vi "Photostimulation engine.vi"(8 "external trigger enabled?":bool, 9 "waveform repetitions":dbl, 10 "pockels and piezo data in":waveform(dbl)[](array[waveform]), 11 "x-y mirror data in":waveform(dbl)[](array[waveform])) -> ()   [LabVIEW 2012]
uses:
  <vilib>/DAQmx/write.llb/DAQmx Write (Analog 1D Wfm NChan NSamp).vi
  <vilib>/Waveform/WDTOps.llb/WDT Number of Waveform Samples DBL.vi
  <vilib>/DAQmx/create/channels.llb/DAQmx Create Channel (AO-Voltage-Basic).vi
  <vilib>/DAQmx/configure/trigger.llb/DAQmx Start Trigger (Digital Edge).vi
  <vilib>/DAQmx/miscellaneous.llb/DAQmx Fill In Error Info.vi
  <resource>/objmgr/daqmx.rc
panel:
  out "String 3":string
  in  "stop 3":bool
  in  "stop 2":bool
  out "Waveform Graph 2":waveform(dbl)[](graph)
  out "Waveform Graph":waveform(dbl)[](graph)
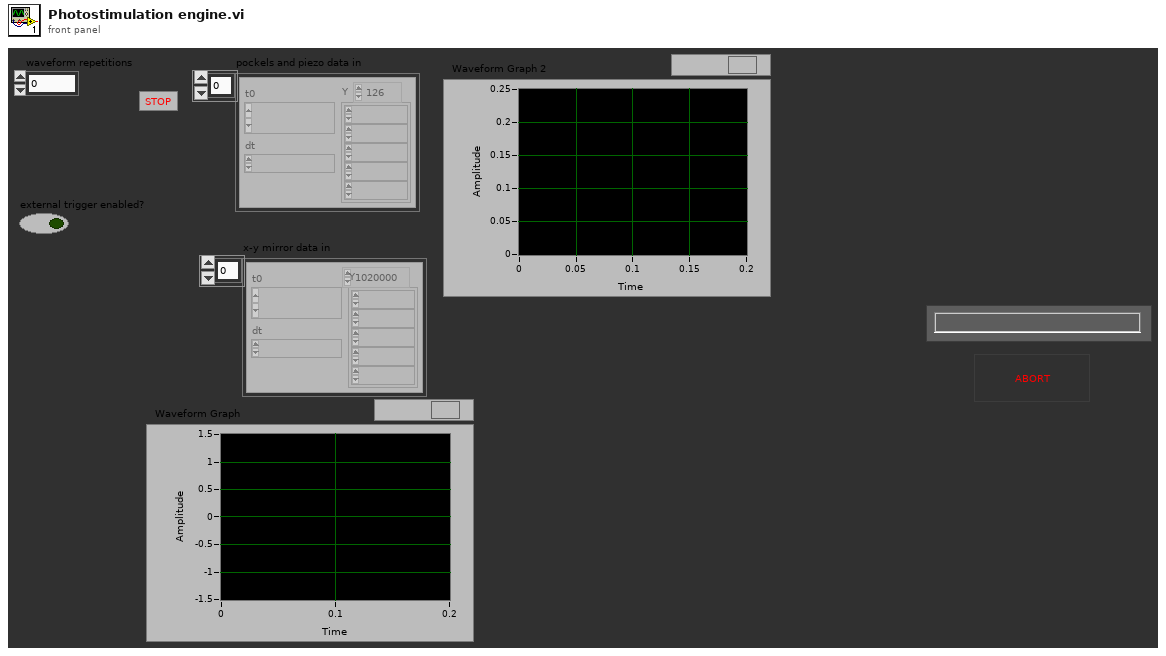
[diagram p1: front panel]
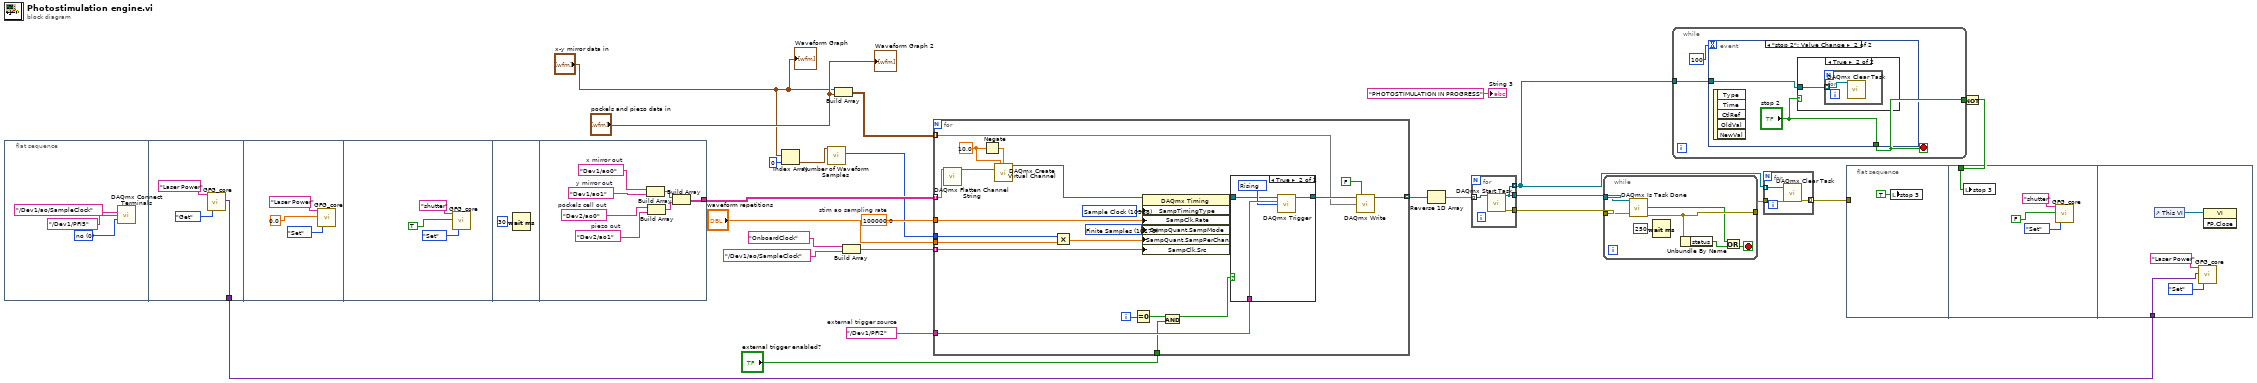
[diagram p0: block diagram]
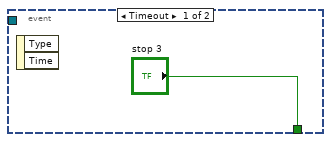
[diagram p2: hidden frame]
diagram:
  w20 = 100000.0  # stim ao sampling rate
  w17 = tag "/Dev1/PFI2"  # external trigger source
  n1 = flat-sequence {
    tunnel: [w29] -> w1
    tunnel: [w39] -> w22
    frame #0 {
      w26 = 0 items=["no", "yes"] ("invert polarity")
      n2 = call <vilib>:"DAQmx Connect Terminals.vi"("source terminal"=tag "/Dev1/ao/SampleClock", "destination terminal"=tag "/Dev1/PFI5", "invert polarity"=w26) -> ()  [unwired: 12 in, 1 out]
    }
    frame #1 {
      n3 = call "GFG_core.vi"("Variable Name in"="Laser Power", "Action"=enum16{"Init", "Set", "Get", "Clear"}."Get") -> ("Variant Out"=w29:variant)  [unwired: 11 in, 6 out]
    }
    frame #2 {
      n4 = call "GFG_core.vi"("Variable Name in"="Laser Power", "Variant in"=0.0 ("waveform repetitions"), "Action"=enum16{"Init", "Set", "Get", "Clear"}."Set") -> ()  [unwired: 10 in, 7 out]
    }
    frame #3 {
      n5 = call "GFG_core.vi"("Variable Name in"="shutter", "Variant in"=TRUE ("external trigger enabled?"), "Action"=enum16{"Init", "Set", "Get", "Clear"}."Set") -> ()  [unwired: 10 in, 7 out]
    }
    frame #4 {
      n6 = Wait (ms)(milliseconds to wait=u32 30) -> ()  [unwired: 1 out]
    }
    frame #5 {
      w42 = tag "Dev2/ao1"  # piezo out
      w43 = tag "Dev2/ao0"  # pockels cell out
      w45 = tag "Dev1/ao1"  # y mirror out
      w44 = tag "Dev1/ao0"  # x mirror out
      n7 = Build Array(w44, w45) -> (w40:tag[])
      n8 = Build Array(w43, w42) -> (w41:tag[])
      n9 = Build Array(w40, w41) -> (w39:tag[][])
    }
  }
  n10 = Index Array(array="x-y mirror data in", index=0) -> (element=w10:waveform(dbl))
  n11 = call-poly <vilib>:"Number of Waveform Samples.vi"("waveform in"=w10) -> ("number of samples"=w9:i32)  [unwired: 8 in, 2 out]
  n12 = Build Array("x-y mirror data in", "pockels and piezo data in") -> (w21:waveform(dbl)[][])
  n13 = Build Array(tag "OnboardClock" ("SampClk.Src"), tag "/Dev1/ao/SampleClock" ("SampClk.Src")) -> (w23:tag[])
  n14 = for {
    tunnel: w22 -> [w58] mode=indexing
    tunnel: w20 -> [w64]
    tunnel: w21 -> [w47] mode=indexing
    tunnel: w17 -> [w63]
    tunnel: w23 -> [w50] mode=indexing
    tunnel: [w56] -> w19 mode=indexing
    tunnel: "external trigger enabled?" -> [w52]
    tunnel: "waveform repetitions" -> [w49]
    tunnel: w9 -> [w46]
    i -> [w55]
    w60 = 10388 items=["Sample Clock"=10388, "Burst Handshake"=12548, "Handshake"=10389, "Implicit"=10451, "On Demand"=10390, "Change Detection"=12504, "Pipelined Sample Clock"=14668] ("SampTimingType")
    w61 = 10178 items=["Finite Samples"=10178, "Continuous Samples"=10123, "Hardware Timed Single Point"=12522] ("SampQuant.SampMode")
    w66 = 10.0 ("maximum value")
    n15 = call <vilib>:"DAQmx Flatten Channel String.vi"("names in"=w58) -> ("names out"=w57:string)  [unwired: 13 in, 1 out]
    n16 = Negate(x=w66) -> (-x=w67:dbl)
    n17 = call-poly <vilib>:"DAQmx Create Virtual Channel.vi"("maximum value"=w66, "minimum value"=w67, "physical channels"=w57) -> ("task out"=w51:refnum<k21>)  [unwired: 11 in, 1 out]
    n18 = Multiply(x=w46, y=w49) -> (x*y=w48:dbl)
    n19 = Equal To 0?(x=w55) -> (x = 0?=w54:bool)
    n20 = property class="DAQmx Timing"(reference=w51, "SampTimingType"=w60, "SampClk.Rate"=w64, "SampQuant.SampMode"=w61, "SampQuant.SampPerChan"=w48, "SampClk.Src"=w50) -> (reference out=w59:refnum<k21>)  [unwired: 1 in, 1 out]
    n21 = And(x=w54, y=w52) -> (x .and. y?=w53:bool)
    n22 = case shown="True" w53 {
      tunnel: w63 -> [_ w72]
      tunnel: [w68 w71] -> w62
      tunnel: w59 -> [w68 w69]
      frame False {
      }
      frame True {
        w70 = 10280 items=["Rising"=10280, "Falling"=10171] ("edge")
        n23 = call-poly <vilib>:"DAQmx Trigger.vi"("task/channels in"=w69, "source"=w72, "edge"=w70) -> ("task out"=w71:refnum<k21>)  [unwired: 11 in, 1 out]
      }
    }
    n24 = call-poly <vilib>:"DAQmx Write.vi"("task/channels in"=w62, "auto start"=FALSE, "data"=w47) -> ("task out"=w56:refnum<k21>)  [unwired: 10 in, 2 out]
  }
  n25 = Reverse 1D Array(array=w19) -> (reversed array=w18:refnum<k21>[])
  n26 = for {
    tunnel: w18 -> [w75] mode=indexing
    tunnel: [w74] -> w14
    tunnel: [w74] -> w3 mode=indexing
    tunnel: [w73] -> w7
    n27 = call <vilib>:"DAQmx Start Task.vi"("task/channels in"=w75) -> ("task out"=w74:refnum<k21>, "error out"=w73:errorcluster)  [unwired: 13 in]
  }
  n28 = while {
    tunnel: w14 -> [w81]
    tunnel: [w79] -> w13
    tunnel: w7 -> [w80]
    stop <- w77 stop-if-true
    n29 = call <vilib>:"DAQmx Is Task Done.vi"("task/channels in"=w81, "error in"=w80) -> ("task done?"=w76:bool, "error out"=w79:errorcluster)  [unwired: 11 in, 1 out]
    n30 = Wait (ms)(milliseconds to wait=u32 250) -> ()  [unwired: 1 out]
    n31 = Unbundle By Name(w79) -> ("status"=w78:bool)
    n32 = Or(x=w76, y=w78) -> (x .or. y?=w77:bool)
  }
  n33 = while {
    tunnel: [w84] -> w5
    tunnel: w3 -> [w83]
    stop <- w84 stop-if-true
    n34 = event shown="[1] \"stop 2\": Value Change" {
      selector: _ -> [_ _]
      dyn-events: _ -> [_ _]
      timeout: 100 -> [_ _]
      tunnel: ["stop 3" "stop 2"] -> w84
      tunnel: w83 -> [_ w87]
      event Timeout {
        n35 = event-data() -> ()  [unwired: 1 in, 2 out]
      }
      event "stop 2": Value Change {
        n36 = event-data() -> ()  [unwired: 1 in, 5 out]
        n37 = case shown="True" "stop 2" {
          tunnel: w87 -> [_ w89]
          frame False {
          }
          frame True {
            n38 = for {
              tunnel: w89 -> [w90] mode=indexing
              n39 = call <vilib>:"DAQmx Clear Task.vi"("task in"=w90) -> ()  [unwired: 14 in, 1 out]
            }
          }
        }
      }
    }
  }
  n40 = for {
    tunnel: w3 -> [w93] mode=indexing
    tunnel: w13 -> [w92]
    tunnel: [w91] -> w6 mode=indexing
    n41 = call <vilib>:"DAQmx Clear Task.vi"("task in"=w93, "error in"=w92) -> ("error out"=w91:errorcluster)  [unwired: 13 in]
  }
  n42 = flat-sequence {
    tunnel: w6 -> [_]
    tunnel: w4 -> [w98]
    tunnel: w1 -> [w99]
    frame #0 {
      n43 = local write "stop 3"(TRUE ("stop 3")) -> ()
    }
    frame #1 {
      n44 = local write "stop 3"(w98) -> ()
      n45 = call "GFG_core.vi"("Variable Name in"="shutter", "Variant in"=FALSE ("external trigger enabled?"), "Action"=enum16{"Init", "Set", "Get", "Clear"}."Set") -> ()  [unwired: 10 in, 7 out]
    }
    frame #2 {
      n46 = control-ref of="This VI"() -> (w102:refnum<vi>)
      n47 = call "GFG_core.vi"("Variable Name in"="Laser Power", "Variant in"=w99, "Action"=enum16{"Init", "Set", "Get", "Clear"}."Set") -> ()  [unwired: 10 in, 7 out]
      n48 = invoke class="VI" method="FP.Close"(reference=w102) -> ()  [unwired: 2 in, 3 out]
    }
  }
  n49 = Not(x=w5) -> (.not. x?=w4:bool)
  "Waveform Graph" <- "x-y mirror data in"
  "Waveform Graph 2" <- "pockels and piezo data in"
  "String 3" <- "PHOTOSTIMULATION IN PROGRESS" ("String 3")
